vi "Log String Message.vi"(8 "Error In":errorcluster, 10 "Message":string, 11 "ILogger In":refnum<class "ILogger.lvclass">) -> (0 "Error Out":errorcluster, 3 "ILogger Out":refnum<class "ILogger.lvclass">)   [LabVIEW 2019, in "ILogger.lvclass"]
uses:
  ILogger.lvclass
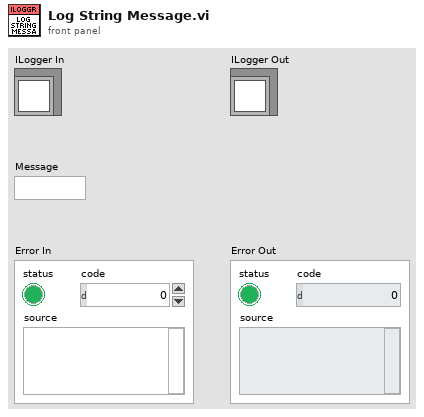
[diagram p1: front panel]
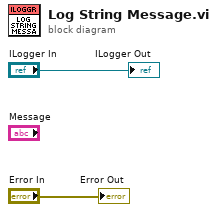
[diagram p0: block diagram]
diagram:
  "Error Out" <- "Error In"
  "ILogger Out" <- "ILogger In"
